vi "Graph_Server_Ready (SubVI).vi"(8 "error in (no error)":errorcluster, 10 "Value":string, 11 "Boolean in":refnum<vi>) -> ()   [LabVIEW 2018]
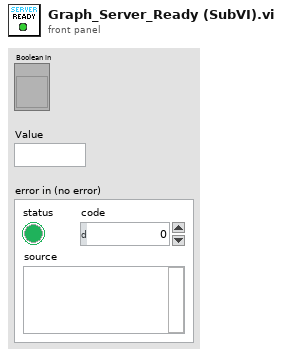
[diagram p1: front panel]
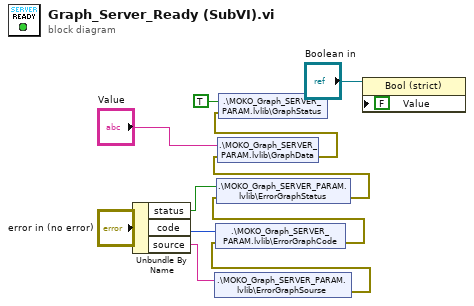
[diagram p0: block diagram]
diagram:
  n1 = Unbundle By Name("error in (no error)") -> ("status"=w8:bool, "code"=w9:i32, "source"=w10:string)
  n2 = shared-variable ".\\MOKO_Graph_SERVER_PARAM.lvlib\\ErrorGraphSourse"(w10) -> (error out=w5:errorcluster)  [unwired: 1 in]
  n3 = shared-variable ".\\MOKO_Graph_SERVER_PARAM.lvlib\\ErrorGraphCode"(w9, error in=w5) -> (error out=w4:errorcluster)
  n4 = shared-variable ".\\MOKO_Graph_SERVER_PARAM.lvlib\\ErrorGraphStatus"(w8, error in=w4) -> (error out=w3:errorcluster)
  n5 = shared-variable ".\\MOKO_Graph_SERVER_PARAM.lvlib\\GraphData"("Value", error in=w3) -> (error out=w2:errorcluster)
  n6 = shared-variable ".\\MOKO_Graph_SERVER_PARAM.lvlib\\GraphStatus"(TRUE, error in=w2) -> ()  [unwired: 1 out]
  n7 = property on="Property Node" class="Bool (strict)"(reference="Boolean in", "Value"=FALSE ("Program busy")) -> ()  [unwired: 1 in, 2 out]
